vi "Query.vi"(8 "error in (no error)":errorcluster, 10 "Command":string, 11 "VISA resource name":refnum<visa-resource-name>) -> (0 "error out":errorcluster, 1 "Resp?":bool, 2 "Response":string, 3 "VISA resource name out":refnum<visa-resource-name>)   [LabVIEW 2019]
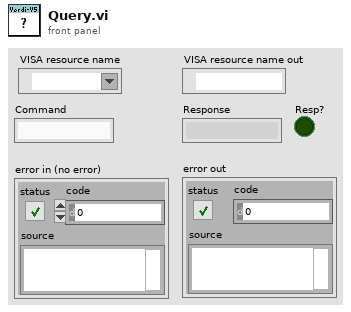
[diagram p1: front panel]
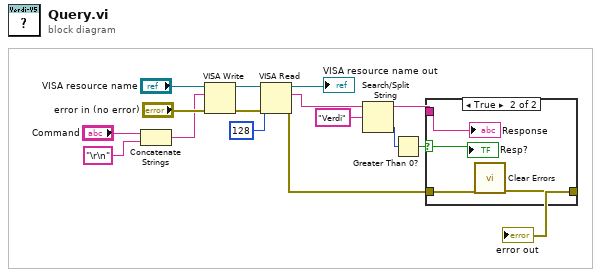
[diagram p0: block diagram]
diagram:
  n1 = Concatenate Strings("Command", "\r\n" ("string")) -> (w14:string)
  n2 = VISA Write(VISA resource name="VISA resource name", write buffer=w14, error in (no error)="error in (no error)") -> (VISA resource name out=w10:refnum<visa-resource-name>, error out=w11:errorcluster)  [unwired: 1 out]
  n3 = VISA Read(VISA resource name=w10, byte count=u32 128, error in (no error)=w11) -> (VISA resource name out=→"VISA resource name out":refnum<visa-resource-name>, read buffer=w5:string, error out=w7:errorcluster)  [unwired: 1 out]
  n4 = Search/Split String(string=w5, search string/char (-)="Verdi") -> (substring before match=w3:string, offset of match=w1:i32)  [unwired: 1 in, 1 out]
  n5 = Greater Than 0?(x=w1) -> (x > 0?=w2:bool)
  n6 = case shown="True" w2 {
    selector: w2 -> [_ w18]
    tunnel: w7 -> [w17 w21]
    tunnel: [w17 w20] -> w6
    tunnel: w3 -> [_ w19]
    frame False {
    }
    frame True {
      n7 = call <vilib>:"Clear Errors.vi"("error in (no error)"=w21) -> ("error out"=w20:errorcluster)  [unwired: 5 in, 1 out]
      "Response" <- w19
      "Resp?" <- w18
    }
  }
  "error out" <- w6
